vi "UntitledSubVI.vi"() -> ()   [LabVIEW 2021]
panel:
  in  "Array":dbl[](array[numeric])
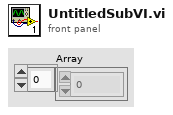
[diagram p1: front panel]
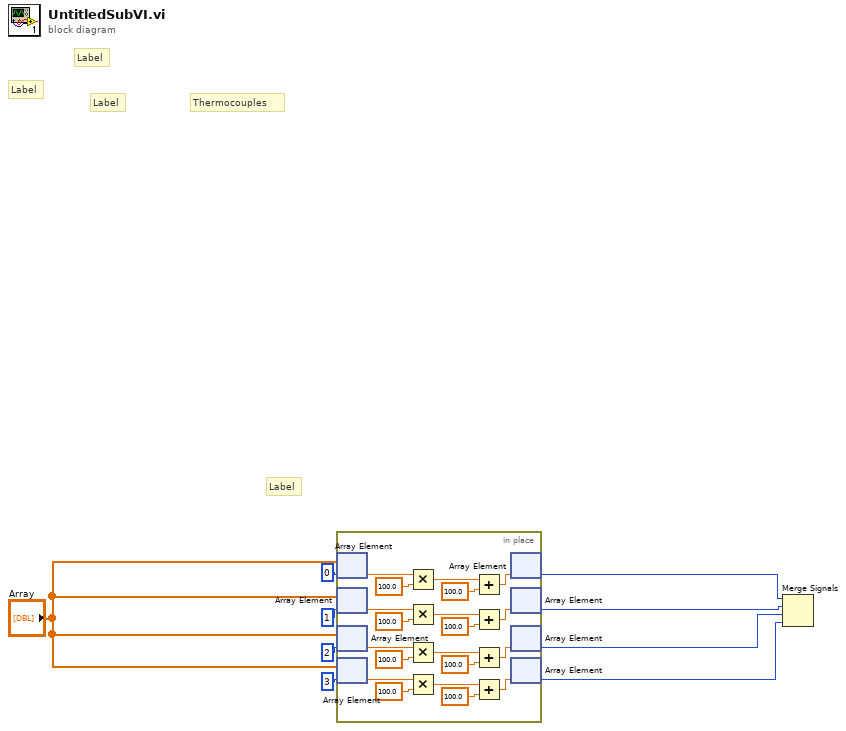
[diagram p0: block diagram]
diagram:
  # "Label"
  # "Label"
  # "Label"
  # "Label"
  # "Thermocouples"
  n1 = in-place {
    n2 = in-place-array #1("Array", 0) -> (w20:dbl)
    n3 = in-place-array #2("Array", 1) -> (w26:dbl)
    n4 = in-place-array #3("Array", 2) -> (w23:dbl)
    n5 = in-place-array #4("Array", 3) -> (w29:dbl)
    n6 = Multiply(x=w20, y=100.0) -> (x*y=w19:dbl)
    n7 = Multiply(x=w26, y=100.0) -> (x*y=w25:dbl)
    n8 = Multiply(x=w23, y=100.0) -> (x*y=w22:dbl)
    n9 = Multiply(x=w29, y=100.0) -> (x*y=w28:dbl)
    n10 = Add(x=w19, y=100.0) -> (x+y=w18:dbl)
    n11 = Add(x=w25, y=100.0) -> (x+y=w24:dbl)
    n12 = Add(x=w22, y=100.0) -> (x+y=w21:dbl)
    n13 = Add(x=w28, y=100.0) -> (x+y=w27:dbl)
    n14 = in-place-array #1(w18) -> (w4:i32)  [unwired: 1 out]
    n15 = in-place-array #2(w24) -> (w3:i32)  [unwired: 1 out]
    n16 = in-place-array #3(w21) -> (w2:i32)  [unwired: 1 out]
    n17 = in-place-array #4(w27) -> (w1:i32)  [unwired: 1 out]
  }
  n18 = Merge Signals(w4, w3, w2, w1) -> ()  [unwired: 1 out]
